vi "Labview3 Convert C to F (JF).vi"() -> ()   [LabVIEW 2023]
panel:
  in  "VISA resource name":refnum<visa-resource-name>
  in  "Temp Scale":bool
  out "Temperature":dbl(slide) scale=0.0..100.0
  # "Deg C"
  # "Deg F"
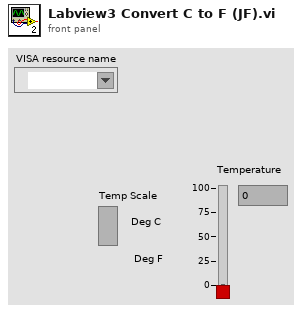
[diagram p1: front panel]
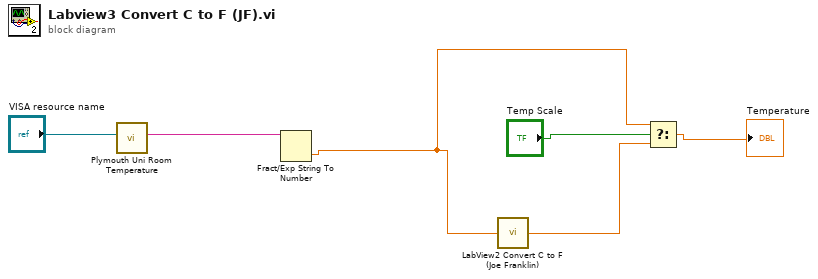
[diagram p0: block diagram]
diagram:
  n1 = call "Plymouth Uni Room Temperature.vi"("VISA resource name"="VISA resource name") -> ("read buffer"=w1:string)  [unwired: 10 in]
  n2 = Fract/Exp String To Number(string=w1) -> (number=w4:dbl)  [unwired: 3 in, 1 out]
  n3 = call "LabView2 Convert C to F (Joe Franklin).vi"("deg (C)"=w4) -> ("deg (F)"=w5:dbl)
  n4 = Select(t=w4, s="Temp Scale", f=w5) -> (s? t:f=→"Temperature":dbl)
